vi "Instrument.Cryostation.getAll.vi"(8 "error in (no error)":errorcluster, 11 "instrument.Cryostation":refnum<class "instrument.Cryostation.lvclass">) -> (0 "error out":errorcluster, 2 "getAll":T1, 3 "instrument.Cryostation out":refnum<class "instrument.Cryostation.lvclass">)   [LabVIEW 2016]
uses:
  instrument.Cryostation.lvclass
  Typedefs/getAll--Cryostation--cluster.ctl
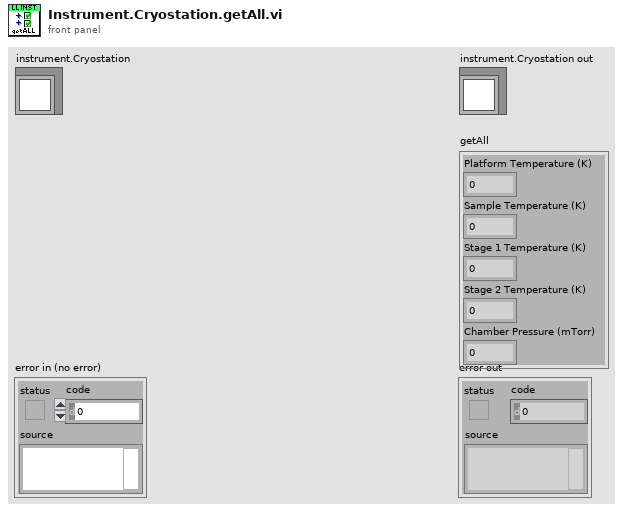
[diagram p1: front panel]
types:
  T1 = typedef "instrument.Cryostation.lvclass/getAll--Cryostation--cluster.ctl" = cluster{"Platform Temperature (K)":dbl, "Sample Temperature (K)":dbl, "Stage 1 Temperature (K)":dbl, "Stage 2 Temperature (K)":dbl, "Chamber Pressure (mTorr)":dbl}
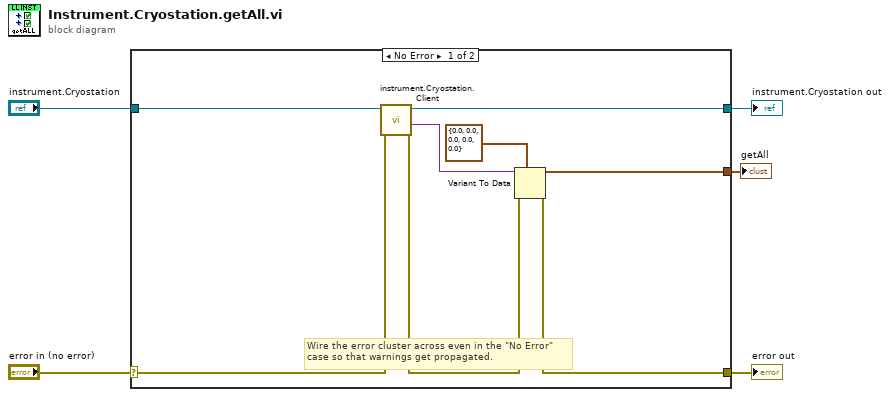
[diagram p0: block diagram]
diagram:
  n1 = case shown="No Error" "error in (no error)" {
    selector: "error in (no error)" -> [w11 w15]
    tunnel: [w9 w15] -> w4
    tunnel: [w12 w14] -> w2
    tunnel: "instrument.Cryostation" -> [w7 w14]
    tunnel: [w8 _] -> w1
    frame No Error {
      # "Wire the error cluster across even in the \"No Error\"\ncase so that warnings get propagated."
      n2 = call "instrument.Cryostation.Client.vi"("error in (no error)"=w11, "instrument.Cryostation in"=w7) -> ("error out"=w10:errorcluster, "Data out"=w13:variant, "instrument.Cryostation out"=w12:refnum<class "instrument.Cryostation.lvclass">)  [unwired: 6 in, 1 out]
      n3 = Variant To Data(error in=w10, type=T1 {"Platform Temperature (K)"=0.0, "Sample Temperature (K)"=0.0, "Stage 1 Temperature (K)"=0.0, "Stage 2 Temperature (K)"=0.0, "Chamber Pressure (mTorr)"=0.0} ("getAll"), Variant=w13) -> (data=w8:T1, error out=w9:errorcluster)
    }
    frame Error {
    }
  }
  "error out" <- w4
  "instrument.Cryostation out" <- w2
  "getAll" <- w1
